vi "Autonomous Independent.vi"() -> ()   [LabVIEW 2018]
doc: "This VI is called when autonomous begins, and will automatically be terminated when autonomous ends. You can carry out timed or sensor driven robot movement independently without needing to return to the caller."
uses:
  Classes/StateMachine/StateMachine.lvclass
  <vilib>/Rock Robotics/WPI/Utilities/WPI_GetSetVariantRefNum.vi
  <vilib>/Rock Robotics/Network Tables/NT Read String.vi
  <vilib>/Rock Robotics/Network Tables/NT Write Numeric Array.vi
  <vilib>/Rock Robotics/WPI/RobotDrive/WPI_RobotDriveArcadeDrive_Standard(NoSaturation).vi
panel:
  out "Numeric":i32
  in  "stop":bool
  out "Current Movement, for debugging":T1 {"Y Joystick Value" scale=1.0..-1.0; "X Joystick Value" scale=-1.0..1.0}
  in  "Array of robot movements":T2(array[cluster])=[{"X Joystick Value"=0.39393939393939403, "Y Joystick Value"=0.0, "Delay (sec)"=1.0, "Movement Name"="turn"}, {"X Joystick Value"=-0.3737373737373737, "Y Joystick Value"=0.0, "Delay (sec)"=1.0, "Movement Name"="turn back"}] {"Y Joystick Value" scale=1.0..-1.0; "X Joystick Value" scale=-1.0..1.0}
  # "Be sure to right-click and choose Data Operations>>Make Current Value default if you want to save the array values with the VI"
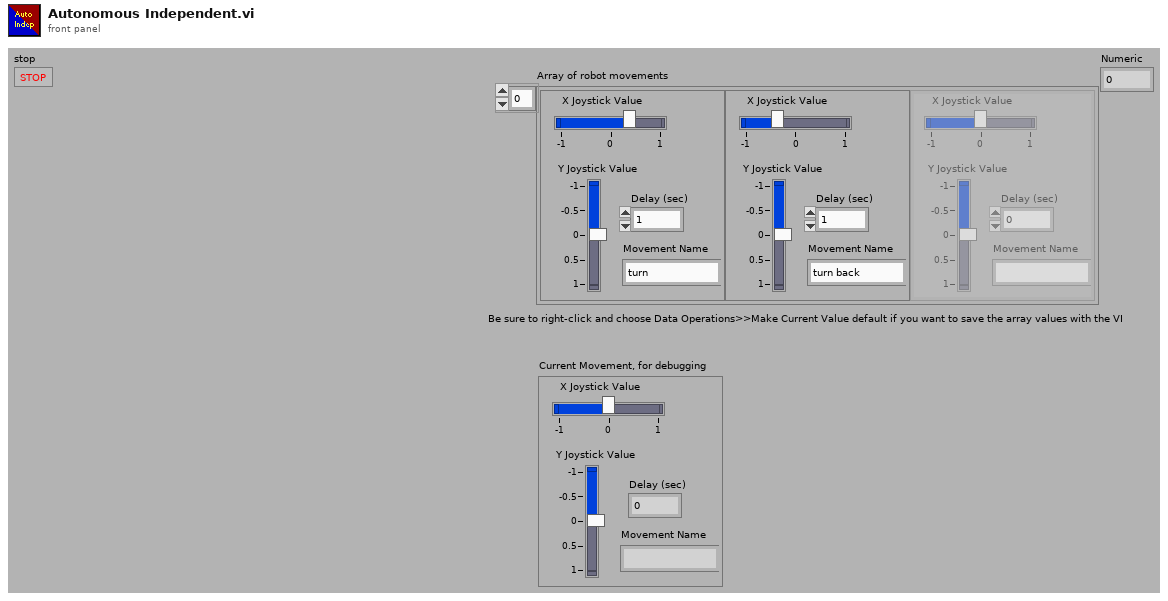
[diagram p1: front panel]
types:
  T1 = cluster{"X Joystick Value":dbl, "Y Joystick Value":dbl, "Delay (sec)":dbl, "Movement Name":string}
  T2 = cluster{"X Joystick Value":dbl, "Y Joystick Value":dbl, "Delay (sec)":dbl, "Movement Name":string}[]
  T3 = typedef "WPI_JoystickDevRef.ctl" = cluster{"Device":T4}
  T4 = typedef "WPI_JoystickDeviceEnum.ctl" = enum16{"USB 0", "USB 1", "USB 2", "USB 3", "USB 4", "USB 5"}
  T5 = cluster{"Run Motionprofile?":bool, "Run Lift?":bool, "Run Vision?":bool, "Run Hatch Outtake?":bool, "Run Hatch Intake?":bool, "Which LiftLevel?":string, "Which MotionProfile?":dbl}
  T6 = typedef "WPI_RobotDriveDevRef.ctl" = cluster{"DevStatus":errorcluster, "Motors[]":T7[], "Square Inputs":bool, "Max Output":dbl}
  T7 = typedef "WPI_MotorControlDeviceRef.ctl" = cluster{"DeviceStatus":errorcluster, "Type":T8, "PWM":cluster{"PWM Channel":T9, "DeadBand":T10}, "CAN":cluster{"Device Number":u8, "SetOutput VI Ref":variant, "GetOutput VI Ref":variant, "Enable VI Ref":variant, "Disable VI Ref":variant, "Data":variant}, "Invert":bool, "DIO PWM":cluster{"PWM \"Enable\" Channel":T9, "DIOChannel":T11, "PWM Rate":dbl}}
  T8 = typedef "WPI_MotorControlType.ctl" = enum16{"PWM", "CAN", "DIO PWM"}
  T9 = typedef "FPGA_DIOPWMChannel.ctl" = enum8{"PWM 0", "PWM 1", "PWM 2", "PWM 3", "PWM 4", "PWM 5", "PWM 6", "PWM 7", "PWM 8", "PWM 9", "PWM MXP 0", "PWM MXP 1", "PWM MXP 2", "PWM MXP 3", "PWM MXP 4", "PWM MXP 5", "PWM MXP 6", "PWM MXP 7", "PWM MXP 8", "PWM MXP 9", "Invalid"}
  T10 = typedef "WPI_PWMDeadband.ctl" = cluster{"Name":string, "maxPositivePwm":i32, "minPositivePwm":i32, "centerPwm":i32, "maxNegativePwm":i32, "minNegativePwm":i32, "angularRange":u16}
  T11 = typedef "FPGA_DIOChannel.ctl" = enum8{"DIO 0", "DIO 1", "DIO 2", "DIO 3", "DIO 4", "DIO 5", "DIO 6", "DIO 7", "DIO 8", "DIO 9", "DIO MXP 0", "DIO MXP 1", "DIO MXP 2", "DIO MXP 3", "DIO MXP 4", "DIO MXP 5", "DIO MXP 6", "DIO MXP 7", "DIO MXP 8", "DIO MXP 9", "DIO MXP 10", "DIO MXP 11", "DIO MXP 12", "DIO MXP 13", "DIO MXP 14", "DIO MXP 15", "SPI Port CS1", "SPI Port CS2", "SPI Port CS3", "SPI Port MISO", "SPI Port MOSI", "Invalid"}
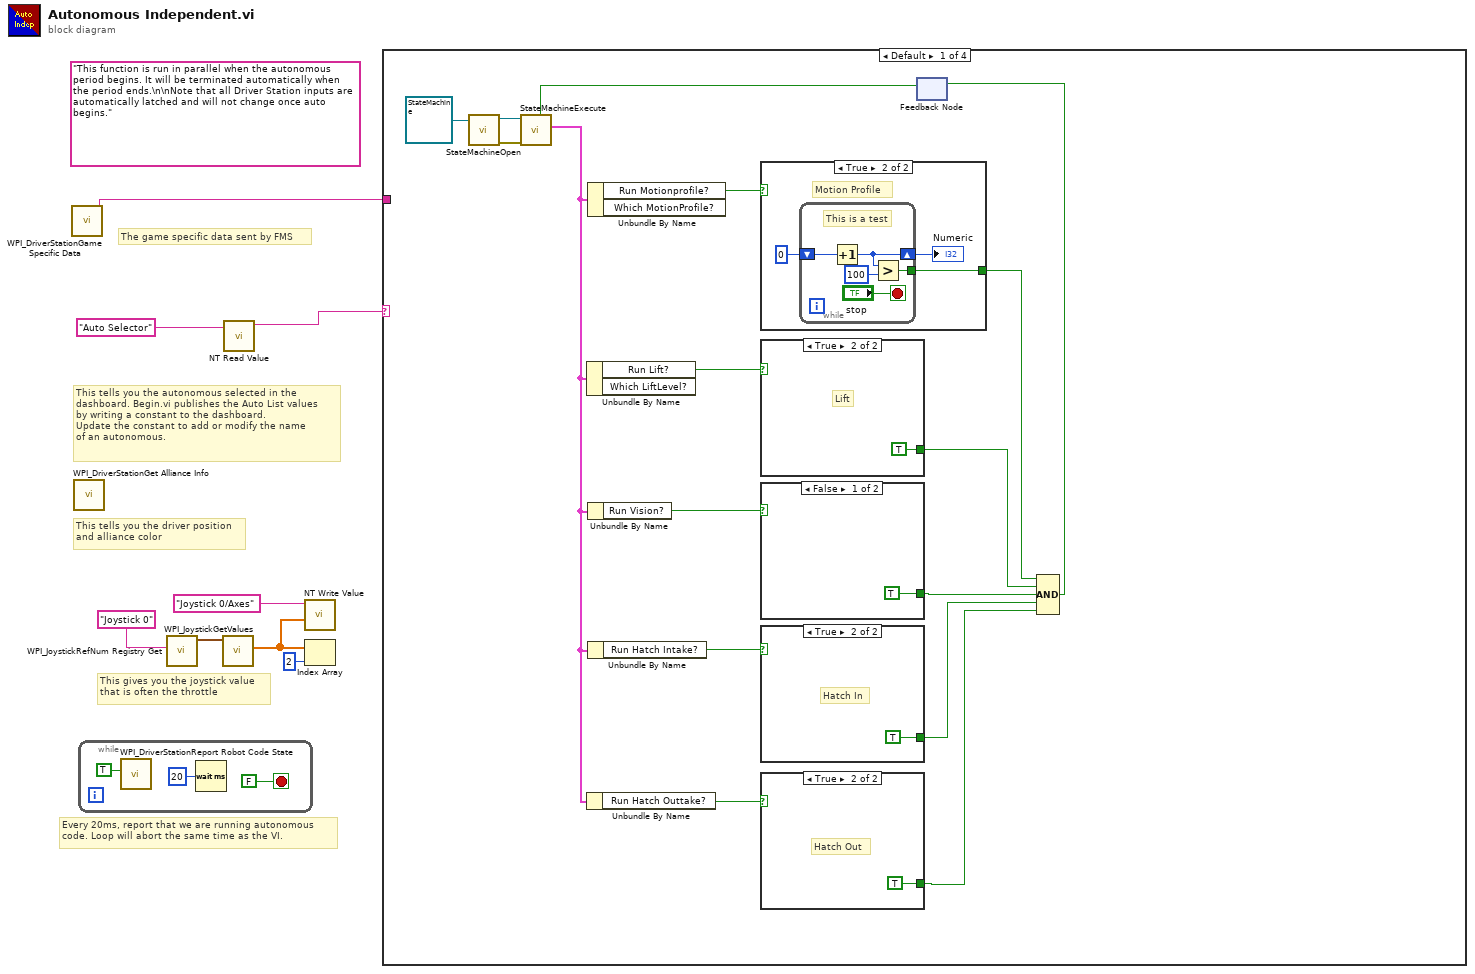
[diagram p0: block diagram]
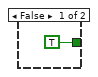
[diagram p2: hidden frame]
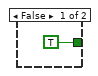
[diagram p3: hidden frame]
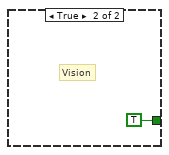
[diagram p4: hidden frame]
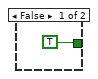
[diagram p5: hidden frame]
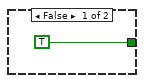
[diagram p6: hidden frame]
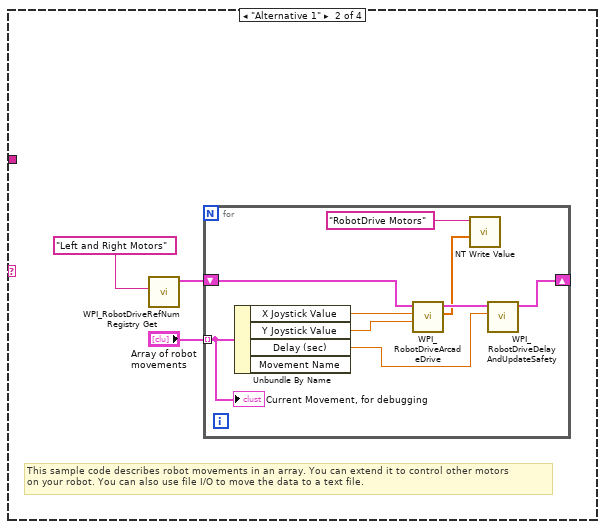
[diagram p7: hidden frame]
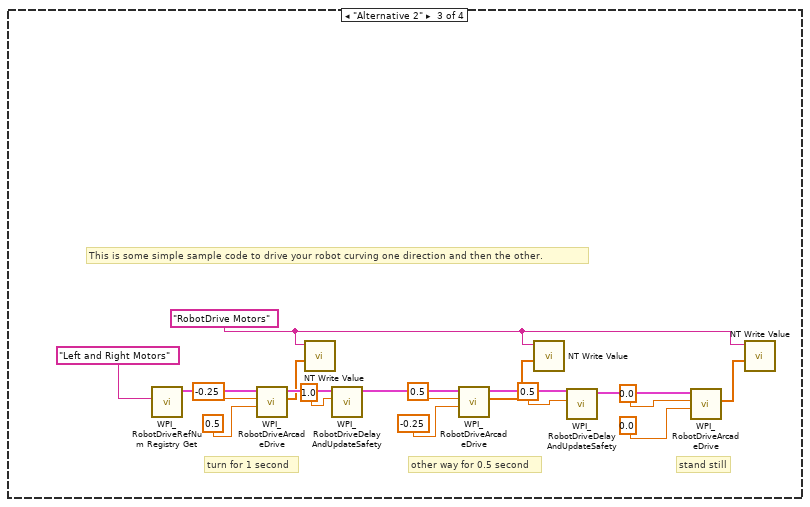
[diagram p8: hidden frame]
diagram:
  (unwired) "This function is run in parallel when the autonomous period begins. It will be terminated automatically when the period ends.\n\nNote that all Driver Station inputs are automatically latched and will not change once auto begins."
  # "The game specific data sent by FMS"
  # "This tells you the autonomous selected in the \ndashboard. Begin.vi publishes the Auto List values\nby writing a constant to the dashboard.\nUpdate the constant to add or modify the name\nof an autonomous."
  # "Every 20ms, report that we are running autonomous\ncode. Loop will abort the same time as the VI."
  # "This gives you the joystick value\nthat is often the throttle"
  # "This tells you the driver position\nand alliance color"
  n1 = call <vilib>:"WPI_DriverStationGame Specific Data.vi"() -> ("Game Specific Data"=w1:string)  [unwired: 11 in]
  n2 = call <vilib>:"WPI_DriverStationGet Alliance Info.vi"() -> ()  [unwired: 12 out]
  n3 = while {
    stop <- FALSE stop-if-true
    n4 = call <vilib>:"WPI_DriverStationReport Robot Code State.vi"("Autonomous"=TRUE) -> ()  [unwired: 10 in, 1 out]
    n5 = Wait (ms)(milliseconds to wait=u32 20) -> ()  [unwired: 1 out]
  }
  n6 = call <vilib>:"WPI_JoystickRefNum Registry Get.vi"("refnum name"="Joystick 0") -> ("JoystickDevRef"=w7:T3)  [unwired: 1 in, 9 out]
  n7 = call <vilib>:"WPI_JoystickGetValues.vi"("JoystickDevRef"=w7) -> ("Axes"=w3:dbl[])  [unwired: 6 in, 4 out]
  n8 = call-poly <vilib>:"NT Read Value.vi"("Name"="Auto Selector") -> ("String"=w4:string)  [unwired: 9 in, 1 out]
  n9 = call-poly <vilib>:"NT Write Value.vi"("Numeric Array"=w3, "Name"="Joystick 0/Axes") -> ()  [unwired: 9 in, 1 out]
  n10 = Index Array(array=w3, index=2) -> ()  [unwired: 1 out]
  n11 = case shown="Default" w4 {
    tunnel: w1 -> [_ _ _ _]
    frame Default {
      n12 = call "StateMachineOpen.vi"("StateMachine in"=refnum<class "StateMachine.lvclass"> refnum ("StateMachine.lvclass")) -> ("error out"=w19:errorcluster, "StateMachine out"=w20:refnum<class "StateMachine.lvclass">)  [unwired: 9 in]
      n13 = feedback #1() -> (w12:bool)  [unwired: 1 in]
      n14 = call "StateMachineExecute.vi"("States finished?"=w12, "error in (no error)"=w19, "StateMachine in"=w20) -> ("output cluster"=w22:T5)  [unwired: 6 in, 2 out]
      n15 = Unbundle By Name(w22) -> ("Run Lift?"=w26:bool)  [unwired: 1 out]
      n16 = Unbundle By Name(w22) -> ("Run Hatch Outtake?"=w23:bool)
      n17 = Unbundle By Name(w22) -> ("Run Motionprofile?"=w27:bool)  [unwired: 1 out]
      n18 = Unbundle By Name(w22) -> ("Run Vision?"=w25:bool)
      n19 = Unbundle By Name(w22) -> ("Run Hatch Intake?"=w24:bool)
      n20 = case shown="True" w27 {
        tunnel: [TRUE w37] -> w18
        frame False {
        }
        frame True {
          # "Motion Profile"
          n21 = while {
            shift-right: [w42] -> w38
            shift-left: 0 -> [w43]
            tunnel: [w40] -> w37
            stop <- "stop" stop-if-true
            # "This is a test"
            n22 = Increment(x=w43) -> (x+1=w42:i32)
            n23 = Greater?(x=w42, y=100) -> (0:w40:bool)
          }
          "Numeric" <- w38
        }
      }
      n24 = case shown="True" w26 {
        tunnel: [TRUE TRUE] -> w17
        frame False {
        }
        frame True {
          # "Lift"
        }
      }
      n25 = case shown="False" w25 {
        tunnel: [TRUE TRUE] -> w16
        frame False {
        }
        frame True {
          # "Vision"
        }
      }
      n26 = case shown="True" w24 {
        tunnel: [TRUE TRUE] -> w15
        frame False {
        }
        frame True {
          # "Hatch In"
        }
      }
      n27 = case shown="True" w23 {
        tunnel: [TRUE TRUE] -> w14
        frame False {
        }
        frame True {
          # "Hatch Out"
        }
      }
      n28 = Compound Arithmetic op=AND(w18, w17, w16, w15, w14) -> (w13:bool)
      n29 = feedback-in #1(w13) -> ()
    }
    frame "Alternative 1" {
      # "This sample code describes robot movements in an array. You can extend it to control other motors\non your robot. You can also use file I/O to move the data to a text file."
      n30 = call <vilib>:"WPI_RobotDriveRefNum Registry Get.vi"("refnum name"="Left and Right Motors") -> ("RobotDriveDevRef"=w46:T6)  [unwired: 1 in, 9 out]
      n31 = for {
        shift-right: [w54] -> _
        shift-left: w46 -> [w55]
        tunnel: "Array of robot movements" -> [w50] mode=indexing
        n32 = Unbundle By Name(w50) -> ("X Joystick Value"=w53:dbl, "Y Joystick Value"=w52:dbl, "Delay (sec)"=w51:dbl)  [unwired: 1 out]
        n33 = call-poly <vilib>:"WPI_RobotDriveArcadeDrive.vi"("Y axis value"=w52, "X axis value"=w53, "RobotDriveDevRef"=w55) -> ("Motor Values"=w48:dbl[], "RobotDriveDevRef"=w56:T6)  [unwired: 1 in, 6 out]
        n34 = call-poly <vilib>:"NT Write Value.vi"("Numeric Array"=w48, "Name"="RobotDrive Motors") -> ()  [unwired: 9 in, 1 out]
        n35 = call <vilib>:"WPI_RobotDriveDelayAndUpdateSafety.vi"("Delay (s)"=w51, "RobotDriveDevRef"=w56) -> ("RobotDriveDevRef 2"=w54:T6)  [unwired: 8 in, 1 out]
        "Current Movement, for debugging" <- w50
      }
    }
    frame "Alternative 2" {
      w58 = "RobotDrive Motors" ("Name")
      # "This is some simple sample code to drive your robot curving one direction and then the other."
      # "stand still"
      # "other way for 0.5 second"
      # "turn for 1 second"
      n36 = call <vilib>:"WPI_RobotDriveRefNum Registry Get.vi"("refnum name"="Left and Right Motors") -> ("RobotDriveDevRef"=w74:T6)  [unwired: 1 in, 9 out]
      n37 = call-poly <vilib>:"WPI_RobotDriveArcadeDrive.vi"("Y axis value"=0.5 ("X axis value"), "X axis value"=-0.25, "RobotDriveDevRef"=w74) -> ("Motor Values"=w57:dbl[], "RobotDriveDevRef"=w67:T6)  [unwired: 1 in, 6 out]
      n38 = call-poly <vilib>:"NT Write Value.vi"("Numeric Array"=w57, "Name"=w58) -> ()  [unwired: 9 in, 1 out]
      n39 = call <vilib>:"WPI_RobotDriveDelayAndUpdateSafety.vi"("Delay (s)"=1.0, "RobotDriveDevRef"=w67) -> ("RobotDriveDevRef 2"=w68:T6)  [unwired: 8 in, 1 out]
      n40 = call-poly <vilib>:"WPI_RobotDriveArcadeDrive.vi"("Y axis value"=-0.25 ("X axis value"), "X axis value"=0.5, "RobotDriveDevRef"=w68) -> ("Motor Values"=w59:dbl[], "RobotDriveDevRef"=w69:T6)  [unwired: 1 in, 6 out]
      n41 = call-poly <vilib>:"NT Write Value.vi"("Numeric Array"=w59, "Name"=w58) -> ()  [unwired: 9 in, 1 out]
      n42 = call <vilib>:"WPI_RobotDriveDelayAndUpdateSafety.vi"("Delay (s)"=0.5, "RobotDriveDevRef"=w69) -> ("RobotDriveDevRef 2"=w70:T6)  [unwired: 8 in, 1 out]
      n43 = call-poly <vilib>:"WPI_RobotDriveArcadeDrive.vi"("Y axis value"=0.0 ("X axis value"), "X axis value"=0.0, "RobotDriveDevRef"=w70) -> ("Motor Values"=w60:dbl[])  [unwired: 1 in, 7 out]
      n44 = call-poly <vilib>:"NT Write Value.vi"("Numeric Array"=w60, "Name"=w58) -> ()  [unwired: 9 in, 1 out]
    }
    frame "Your Turn" {
    }
  }
